vi "E710_Simple_Test.vi"(0 "System no.":i32=1 min=1 step=1, 5 "error in":errorcluster, 6 "Interface":u16(ring) items=["RS232", "GPIB"], 7 "Timeout":u32=5000, 8 "RS232 settings":cluster{"Portnumber":i32, "Baudrate":u16}={"Portnumber"=0, "Baudrate"=4} {"Baudrate" items=["9600", "14400", "19200", "38400", "57600", "115200"]; "Portnumber" items=["COM1", "COM2", "COM3", "COM4", "COM5", "COM6", "COM7", "COM8", "COM9", "COM10", "COM11", "COM12", "COM13", "COM14", "COM15", "COM16", "COM17", "COM18", "COM19", "COM20", "COM21", "COM22", "COM23", "COM24", "COM25", "COM26", "COM27", "COM28", "COM29", "COM30"]}, 9 "GPIB settings":cluster{"Bus":i32, "Address":i32}={"Bus"=0, "Address"=4}) -> (14 "Identification":string, 16 "Axis IDs":string[](array[string]), 19 "error out":errorcluster)   [LabVIEW 2011]
doc: "This simple test VI is a stand-alone sample application. Use the \nHelp - Show Context Help menu sequence in the LabVIEW environment to display the Context Help window with the control/indicator descriptions.\nSpecify \nØ System no. (= 1 in a one-system configuration),\nØ Interface (= RS232 or GPIB)\nØ Timeout value (in milliseconds)\nØ and interface settings first.\nThen start the VI. The VI will open a connection to the E-710 and query the controller for its identification string and the available axis IDs. The diagram shows how to combine the driver and support VIs for these tasks."
uses:
  Low Level/Communication.llb/Global1.vi
panel:
  # "Simple E-710 communication test program"
  # "Select E-710 interface, timeout value and interface settings first, then start the VI. The VI will open the chosen port, query for \nthe available axis IDs and query for Identification (*IDN?). See VI and control/ indicator information for details."
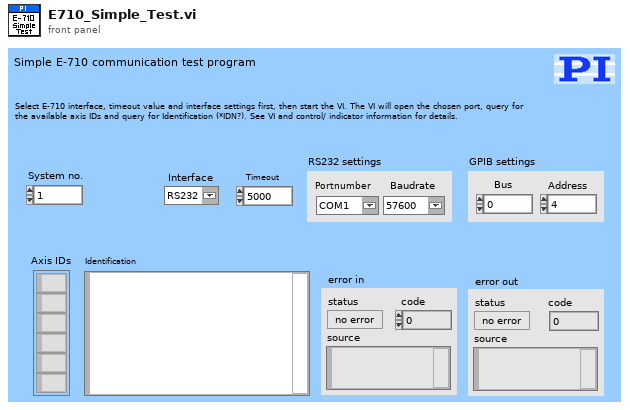
[diagram p1: front panel]
types:
  T1 = typedef "Available DLLs.ctl" = u16
  T2 = typedef "Available DLL interfaces.ctl" = u16
  T3 = cluster{"DLL for Device":T1, "DLL Interface":T2, "Parameter":string}[]
  T4 = typedef "Available interfaces.ctl" = u16
  T5 = cluster{"RS232 Portnumber":i32, "Timeout":i32, "RS232 Baud rate":u32, "Interface":T4, "GPIB Bus":i32, "GPIB Address":i32, "GPIB Mode":i32}[]
  T6 = cluster{"input XON/XOFF":bool, "input HW Handshake":bool, "input alt HW HShk":bool, "output XON/XOFF":bool, "output HW Handshake":bool, "output alt HW HShk":bool, "XOFF byte ":u8, "XON byte":u8, "parity error byte":u16}[]
  T7 = cluster{"DLL for Device":T1, "DLL Interface":T2, "Parameter":string}
  T8 = cluster{"RS232 Portnumber":i32, "Timeout":i32, "RS232 Baud rate":u32, "Interface":T4, "GPIB Bus":i32, "GPIB Address":i32, "GPIB Mode":i32}
  T9 = cluster{"input XON/XOFF":bool, "input HW Handshake":bool, "input alt HW HShk":bool, "output XON/XOFF":bool, "output HW Handshake":bool, "output alt HW HShk":bool, "XOFF byte ":u8, "XON byte":u8, "parity error byte":u16}
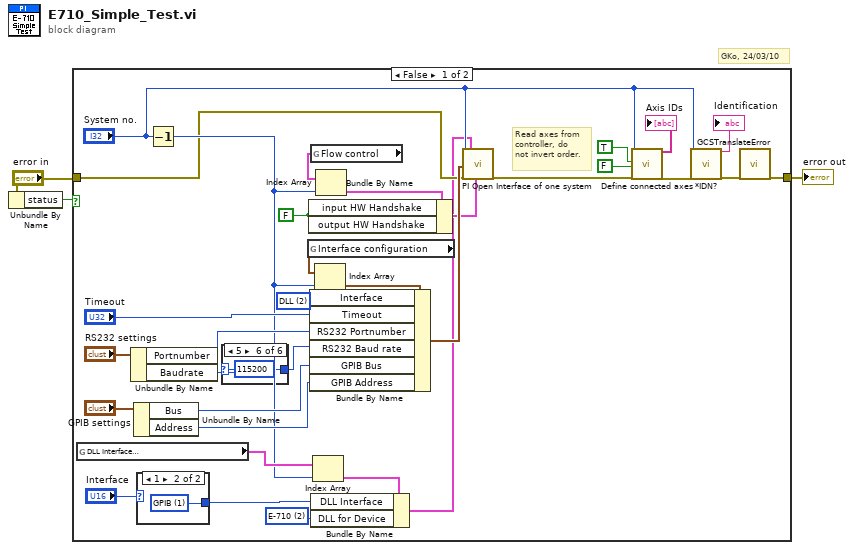
[diagram p0: block diagram]
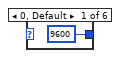
[diagram p2: hidden frame]
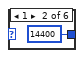
[diagram p3: hidden frame]
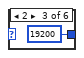
[diagram p4: hidden frame]
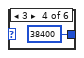
[diagram p5: hidden frame]
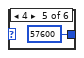
[diagram p6: hidden frame]
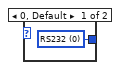
[diagram p7: hidden frame]
diagram:
  # "GKo, 24/03/10"
  n1 = Unbundle By Name("error in") -> ("status"=w1:bool)
  n2 = case shown="False" w1 {
    tunnel: [w4 w45] -> w2
    tunnel: "error in" -> [w8 w45]
    frame False {
      w20 = FALSE ("Bundle Element")
      w9 = u16 2 items=["C-843", "C-844", "E-710", "C-843.PM", "C-865"] ("DLL for Device")
      w14 = u16 2 items=["RS232", "GPIB", "DLL"] ("Interface")
      # "Read axes from\ncontroller, do\nnot invert order."
      n3 = global read "Global1.vi" "DLL Interface\nConfiguration"() -> (w13:T3)
      n4 = Unbundle By Name("RS232 settings") -> ("Portnumber"=w28:i32, "Baudrate"=w27:u16)
      n5 = Unbundle By Name("GPIB settings") -> ("Bus"=w24:i32, "Address"=w23:i32)
      n6 = case shown="1" "Interface" {
        tunnel: [w43 w44] -> w10
        frame 0, Default {
          w43 = u16 0 items=["RS232", "GPIB", "DLL"] ("Interface")
        }
        frame 1 {
          w44 = u16 1 items=["RS232", "GPIB", "DLL"] ("Interface")
        }
      }
      n7 = Decrement(x="System no.") -> (x-1=w11:i32)
      n8 = case shown="5" w27 {
        tunnel: [u32 9600 u32 14400 u32 19200 u32 38400 u32 57600 u32 115200] -> w26
        frame 0, Default {
        }
        frame 1 {
        }
        frame 2 {
        }
        frame 3 {
        }
        frame 4 {
        }
        frame 5 {
        }
      }
      n9 = global read "Global1.vi" "Interface configuration"() -> (w22:T5)
      n10 = global read "Global1.vi" "Flow control"() -> (w19:T6)
      n11 = Index Array(array=w13, index=w11) -> (element=w12:T7)
      n12 = Bundle By Name(cluster=w12, "DLL Interface"=w10, "DLL for Device"=w9) -> (w7:T7)
      n13 = Index Array(array=w22, index=w11) -> (element=w32:T8)
      n14 = Bundle By Name(cluster=w32, "Interface"=w14, "Timeout"="Timeout", "RS232 Portnumber"=w28, "RS232 Baud rate"=w26, "GPIB Bus"=w24, "GPIB Address"=w23) -> (w18:T8)
      n15 = Index Array(array=w19, index=w11) -> (element=w21:T9)
      n16 = Bundle By Name(cluster=w21, "input HW Handshake"=w20, "output HW Handshake"=w20) -> (w17:T9)
      n17 = call "PI Open Interface of one system.vi"("System number"="System no.", "Interface configuration"=w18, "error in"=w8, "DLL Interface\nConfiguration"=w7, "Flow control"=w17) -> ("error out"=w34:errorcluster)  [unwired: 7 in, 7 out]
      n18 = call "Define connected axes.vi"("System no."="System no.", "Read from\ncontroller?"=TRUE ("Read from\nController"), "Invert\norder?"=FALSE ("Invert\norder?"), "error in"=w34) -> ("Conn. Axes out"=→"Axis IDs":string[], "error out"=w16:errorcluster)  [unwired: 1 in, 13 out]
      n19 = call "*IDN?.vi"("System no."="System no.", "error in"=w16) -> ("Identification"=→"Identification":string, "error out"=w5:errorcluster)  [unwired: 16 out]
      n20 = call "GCSTranslateError.vi"("error in"=w5) -> ("error out"=w4:errorcluster)  [unwired: 18 out]
    }
    frame True {
    }
  }
  "error out" <- w2
